vi "Wait For Packet.vi"(8 "Error In":errorcluster, 11 "LINX Device Config":T1) -> (0 "Error Out":errorcluster, 2 "Packet":u8[](array[numeric]), 3 "LINX Device Config":T1)   [LabVIEW 2011, in "LVH-LINX.lvlib"]
doc: "Wait until a LINX return packet is received or a timout occurs. If a valid packet is recieved this VI will return that packet otherwise this VI returns and empty packet and generates an error."
uses:
  LVH-LINX.lvlib
  Type Defs/LINX Device Config.ctl
  Type Defs/Interface.ctl
  Type Defs/TCP Config.ctl
  Error Type.ctl
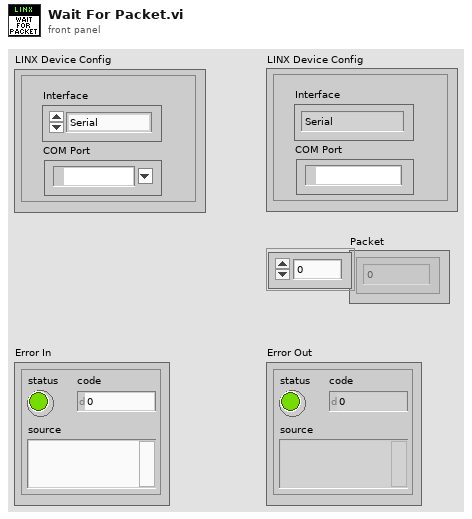
[diagram p1: front panel]
types:
  T1 = typedef "LVH-LINX.lvlib/LINX Device Config.ctl" = cluster{"Interface":T2, "COM Port":refnum<visa-resource-name>, "Packet Number":u16, "TCP Configuration":T3}
  T2 = typedef "LVH-LINX.lvlib/Interface.ctl" = enum16{"Serial", "TCP"}
  T3 = typedef "LVH-LINX.lvlib/TCP Config.ctl" = cluster{"IP Address":string, "Port":dbl}
  T4 = typedef "LVH-LINX.lvlib/Error Type.ctl" = enum16{"Unknown", "Timeout", "Corrupt Return Packet", "Unable To Connect"}
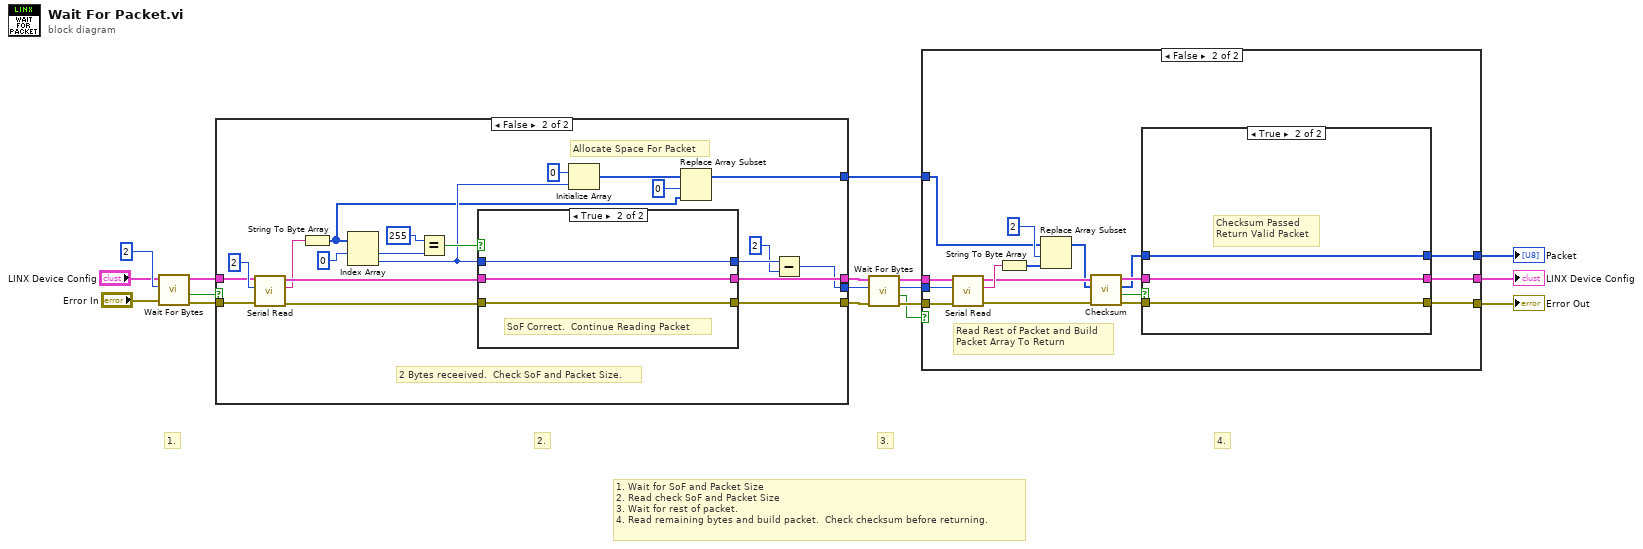
[diagram p0: block diagram]
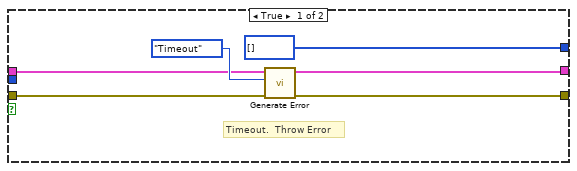
[diagram p2: hidden frame]
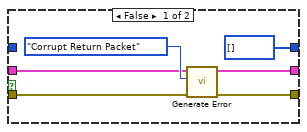
[diagram p3: hidden frame]
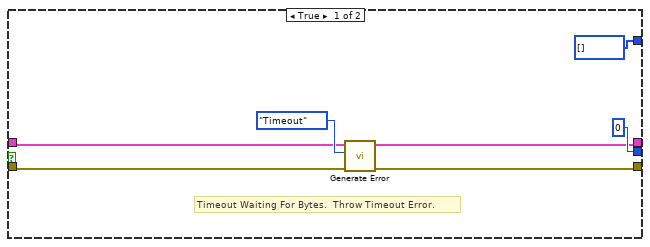
[diagram p4: hidden frame]
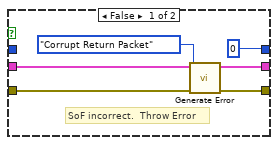
[diagram p5: hidden frame]
diagram:
  # "4."
  # "1. Wait for SoF and Packet Size\n2. Read check SoF and Packet Size\n3. Wait for rest of packet.\n4. Read remaining bytes and build packet.  Check checksum before returning."
  # "3."
  # "2."
  # "1."
  n1 = call "Wait For Bytes.vi"("Error In"="Error In", "Num Bytes"=u32 2, "LINX Device Config"="LINX Device Config") -> ("Error Out"=w16:errorcluster, "Timeout"=w8:bool, "LINX Device Config"=w15:T1)  [unwired: 5 in, 1 out]
  n2 = case shown="False" w8 {
    tunnel: w16 -> [w22 w33]
    tunnel: w15 -> [w18 w31]
    tunnel: [u8 0 w25] -> w13
    tunnel: [w21 w41] -> w11
    tunnel: [w19 w34] -> w12
    tunnel: [u8[] [] w35] -> w5
    frame True {
      # "Timeout Waiting For Bytes.  Throw Timeout Error."
      n3 = call "Generate Error.vi"("Error In"=w22, "Error Type"=Error_Type."Timeout", "LINX Device Config"=w18) -> ("Error Out"=w21:errorcluster, "LINX Device Config"=w19:T1)  [unwired: 7 in]
    }
    frame False {
      # "Allocate Space For Packet"
      # "2 Bytes receeived.  Check SoF and Packet Size."
      n4 = call "Serial Read.vi"("Error In"=w33, "Bytes To Read"=u32 2 ("byte count"), "LINX Device Config"=w31) -> ("Error Out"=w29:errorcluster, "Data"=w28:string, "LINX Device Config"=w30:T1)  [unwired: 6 in]
      n5 = String To Byte Array(string=w28) -> (unsigned byte array=w36:u8[])
      n6 = Index Array(array=w36, index #1=0 ("index")) -> (element #1=w44:u8, element #2=w40:u8)  [unwired: 1 in]
      n7 = Equal?(x=u8 255, y=w44) -> (x = y?=w42:bool)
      n8 = case shown="True" w42 {
        tunnel: w40 -> [_ w52]
        tunnel: w29 -> [w51 w54]
        tunnel: [w50 w54] -> w41
        tunnel: [w47 w53] -> w34
        tunnel: w30 -> [w48 w53]
        tunnel: [u8 0 w52] -> w27
        frame False {
          # "SoF incorrect.  Throw Error"
          n9 = call "Generate Error.vi"("Error In"=w51, "Error Type"=Error_Type."Corrupt Return Packet", "LINX Device Config"=w48) -> ("Error Out"=w50:errorcluster, "LINX Device Config"=w47:T1)  [unwired: 7 in]
        }
        frame True {
          # "SoF Correct.  Continue Reading Packet"
        }
      }
      n10 = Initialize Array(u8 0 ("element"), w40) -> (w38:u8[])
      n11 = Replace Array Subset(array=w38, new element=w36, index=0) -> (w35:u8[])
      n12 = Subtract(x=w27, y=u8 2) -> (x-y=w25:u8)
    }
  }
  n13 = call "Wait For Bytes.vi"("Error In"=w11, "Num Bytes"=w13, "LINX Device Config"=w12) -> ("Error Out"=w10:errorcluster, "Timeout"=w6:bool, "Num Bytes"=w7:u32, "LINX Device Config"=w9:T1)  [unwired: 5 in]
  n14 = case shown="False" w6 {
    tunnel: w10 -> [w59 w72]
    tunnel: w9 -> [w56 w73]
    tunnel: w7 -> [_ w71]
    tunnel: [w58 w75] -> w4
    tunnel: [w55 w74] -> w2
    tunnel: w5 -> [_ w69]
    tunnel: [u8[] [] ("unsigned byte array") w61] -> w3
    frame True {
      # "Timeout.  Throw Error"
      n15 = call "Generate Error.vi"("Error In"=w59, "Error Type"=Error_Type."Timeout", "LINX Device Config"=w56) -> ("Error Out"=w58:errorcluster, "LINX Device Config"=w55:T1)  [unwired: 7 in]
    }
    frame False {
      # "Read Rest of Packet and Build\nPacket Array To Return"
      n16 = call "Serial Read.vi"("Error In"=w72, "Bytes To Read"=w71, "LINX Device Config"=w73) -> ("Error Out"=w68:errorcluster, "Data"=w70:string, "LINX Device Config"=w67:T1)  [unwired: 6 in]
      n17 = String To Byte Array(string=w70) -> (unsigned byte array=w76:u8[])
      n18 = Replace Array Subset(array=w69, new element=w76, index=2) -> (w66:u8[])
      n19 = call "Checksum.vi"("Error In"=w68, "Packet"=w66, "LINX Device Config"=w67) -> ("Error Out"=w64:errorcluster, "Checksum Pass?"=w63:bool, "Packet"=w62:u8[], "LINX Device Config"=w65:T1)  [unwired: 5 in]
      n20 = case shown="True" w63 {
        tunnel: [w83 w86] -> w75
        tunnel: w64 -> [w82 w86]
        tunnel: [w79 w85] -> w74
        tunnel: w65 -> [w80 w85]
        tunnel: w62 -> [_ w84]
        tunnel: [u8[] [] w84] -> w61
        frame False {
          n21 = call "Generate Error.vi"("Error In"=w82, "Error Type"=Error_Type."Corrupt Return Packet", "LINX Device Config"=w80) -> ("Error Out"=w83:errorcluster, "LINX Device Config"=w79:T1)  [unwired: 7 in]
        }
        frame True {
          # "Checksum Passed\nReturn Valid Packet"
        }
      }
    }
  }
  "Error Out" <- w4
  "Packet" <- w3
  "LINX Device Config" <- w2
